vi "apply PID changes.vi"(8 "error in":errorcluster, 9 "new channel":refnum<class "PID Loop.lvclass">, 10 "old channel":refnum<class "PID Loop.lvclass">, 11 "Tagbus PID Module configuration in":refnum<class "Tagbus PID Module configuration.lvclass">) -> (0 "error out":errorcluster, 3 "Tagbus PID Module configuration out":refnum<class "Tagbus PID Module configuration.lvclass">)   [LabVIEW 2014, in "Tagbus PID Module configuration.lvclass"]
uses:
  Tagbus PID Module configuration.lvclass
  PID Loop.lvclass
  Tagbus PID Module configuration.lvclass/Tagbus PID Module configuration.ctl
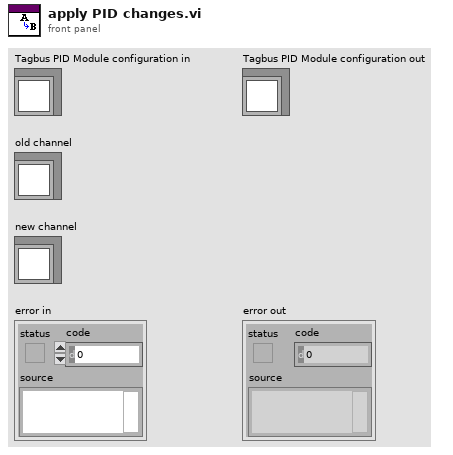
[diagram p1: front panel]
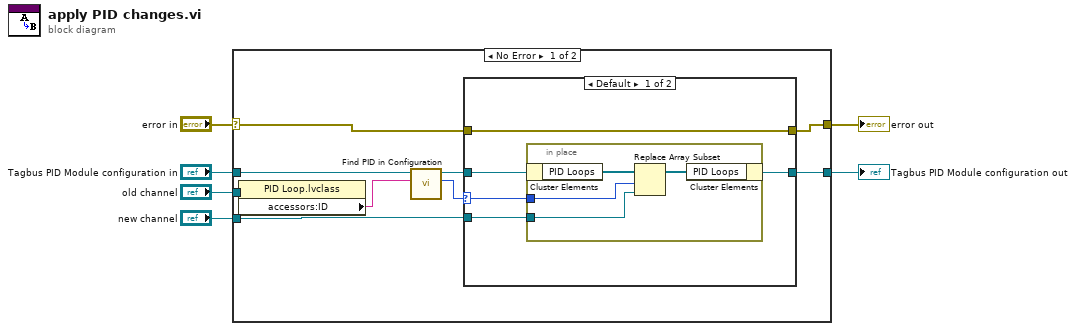
[diagram p0: block diagram]
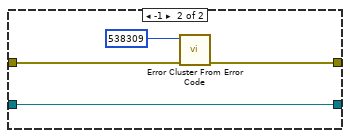
[diagram p2: hidden frame]
diagram:
  n1 = case shown="No Error" "error in" {
    selector: "error in" -> [w14 w30]
    tunnel: [w13 w30] -> w5
    tunnel: [w9 w29] -> w3
    tunnel: "Tagbus PID Module configuration in" -> [w12 w29]
    tunnel: "old channel" -> [w8 _]
    tunnel: "new channel" -> [w15 _]
    frame No Error {
      n2 = property class="PID Loop.lvclass"(reference=w8) -> ("accessors:ID"=w7:string)  [unwired: 1 in, 2 out]
      n3 = call "Find PID in Configuration.vi"("PID Loop ID in"=w7, "Tagbus PID Module configuration in"=w12) -> ("index"=w11:i32, "Tagbus PID Module configuration out"=w10:refnum<class "Tagbus PID Module configuration.lvclass">)  [unwired: 8 in]
      n4 = case shown="Default" w11 {
        selector: w11 -> [w20 _]
        tunnel: w15 -> [w19 _]
        tunnel: w14 -> [w18 w27]
        tunnel: [w18 w26] -> w13
        tunnel: w10 -> [w17 w25]
        tunnel: [w16 w25] -> w9
        frame Default {
          n5 = in-place {
            in-place-border: w20 -> [w24]
            in-place-border: w19 -> [w23]
            n6 = in-place-cluster #1(w17) -> ("PID Loops"=w22:refnum<class "PID Loop.lvclass">[])
            n7 = Replace Array Subset(array=w22, new element=w23, index=w24) -> (w21:refnum<class "PID Loop.lvclass">[])
            n8 = in-place-cluster #1("PID Loops"=w21) -> (w16:refnum<class "Tagbus PID Module configuration.lvclass">)
          }
        }
        frame -1 {
          n9 = call <vilib>:"Error Cluster From Error Code.vi"("error in (no error)"=w27, "error code (0)"=538309) -> ("error out"=w26:errorcluster)  [unwired: 7 in]
        }
      }
    }
    frame Error {
    }
  }
  "error out" <- w5
  "Tagbus PID Module configuration out" <- w3
